vi "Fill FN - Post-Fill Wait (SubVI).vi"(0 "Signals IN":T2={"Dispense"=FALSE, "Fill"=FALSE, "Spray"=FALSE, "Drain"=TRUE, "Complete"=FALSE, "Fill Error"=FALSE, "Dispense Error"=FALSE, "Fill Timeout"=FALSE, "Dispense Timeout"=FALSE}, 1 "Values IN":T1 {"Drain Time (s)" format="%.2f"; "Drain Rate (g/sec)" format="%.2f"}, 2 "Measured Mass (g)":dbl(knob) scale=0.0..1000.0, 3 "Settings":T3={"ON Settings"={"Enable Dynamic Setpoint?"=TRUE, "Enable Dynamic Dispense Time?"=TRUE, "Enable Drain Rate Functions"=TRUE, "Dispense Sample Time (s)"=0.5, "Dispense Slope Ave"=0, "ON Timeout (sec)"=600.0, "1st Setpoint (% of Target)"=0.0, "2nd Setpoint (% of Target)"=0.0, "3rd Setpoint (% of Target)"=0.0, "Measure Dispense Delay (sec)"=0.0, "Settle Slope Sample Time (s)"=0.0}, "OFF Settings"={"Drain Sample Time (s)"=0.5, "Drain Rate Ave Size"=5, "Drain Rate Limits (± g/sec)"=10.0, "Level Slope Range (± g/sec)"=0.25, "OFF Timeout (sec)"=0.0, "Near SP Slope Level (± g/sec)"=0.01, "Near Setpoint Threshold (%)"=95.0}, "Overshoot Settings"={"Time Limit (s)"=60.0, "Container MAX (g)"=1500.0, "Max FILL Slope (+/- g/sec)"=10.0, "% Overshot to Enable (>)"=0.25}, "FILL Timeout (s)"=300.0, "Full Settle Time (s)"=20.0, "Pre-Hydrate \nSpray Time (s)"=10.0, "Pre-Hydrate \nWait Time (s)"=30.0}, 5 "Fill Case Change?":bool) -> (14 "Signals OUT":T2, 15 "Values OUT":T1, 19 "Case Complete":bool)   [LabVIEW 2012]
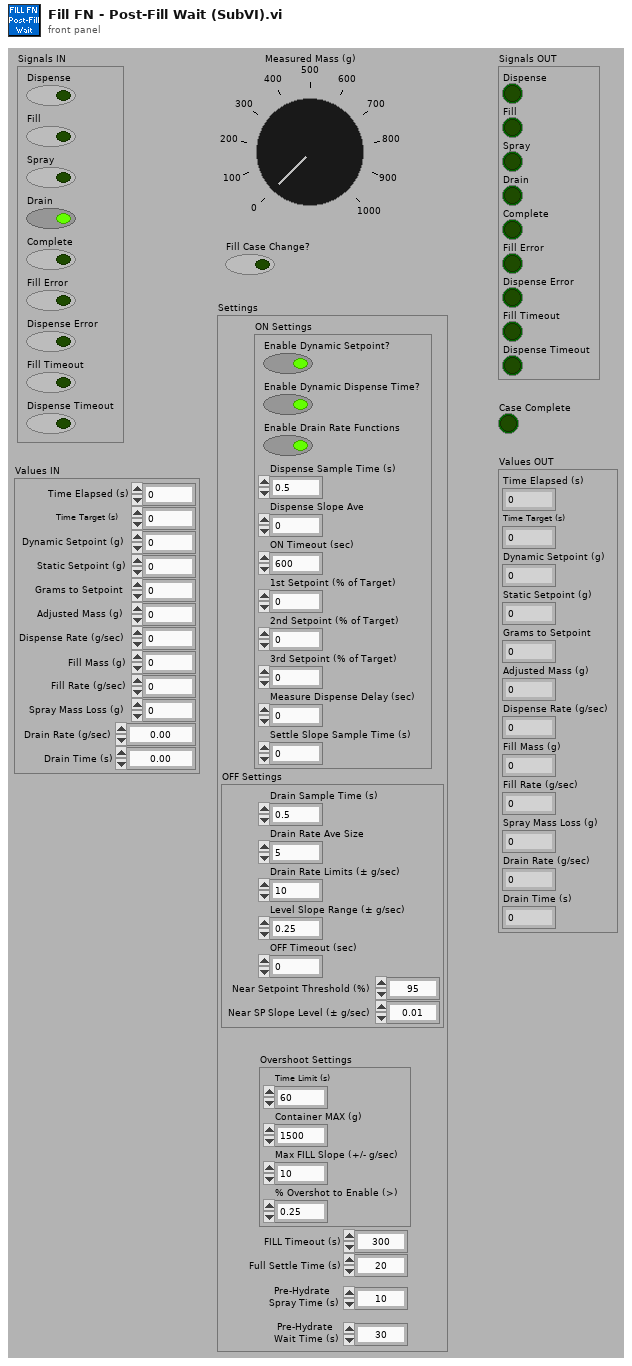
[diagram p1: front panel]
types:
  T1 = cluster{"Time Elapsed (s)":dbl, "Time Target (s)":dbl, "Dynamic Setpoint (g)":dbl, "Static Setpoint (g)":dbl, "Grams to Setpoint":dbl, "Adjusted Mass (g)":dbl, "Dispense Rate (g/sec)":dbl, "Fill Mass (g)":dbl, "Fill Rate (g/sec)":dbl, "Spray Mass Loss (g)":dbl, "Drain Rate (g/sec)":dbl, "Drain Time (s)":dbl}
  T2 = cluster{"Dispense":bool, "Fill":bool, "Spray":bool, "Drain":bool, "Complete":bool, "Fill Error":bool, "Dispense Error":bool, "Fill Timeout":bool, "Dispense Timeout":bool}
  T3 = cluster{"ON Settings":cluster{"Enable Dynamic Setpoint?":bool, "Enable Dynamic Dispense Time?":bool, "Enable Drain Rate Functions":bool, "Dispense Sample Time (s)":dbl, "Dispense Slope Ave":i32, "ON Timeout (sec)":dbl, "1st Setpoint (% of Target)":dbl, "2nd Setpoint (% of Target)":dbl, "3rd Setpoint (% of Target)":dbl, "Measure Dispense Delay (sec)":dbl, "Settle Slope Sample Time (s)":dbl}, "OFF Settings":cluster{"Drain Sample Time (s)":dbl, "Drain Rate Ave Size":i32, "Drain Rate Limits (± g/sec)":dbl, "Level Slope Range (± g/sec)":dbl, "OFF Timeout (sec)":dbl, "Near SP Slope Level (± g/sec)":dbl, "Near Setpoint Threshold (%)":dbl}, "Overshoot Settings":cluster{"Time Limit (s)":dbl, "Container MAX (g)":dbl, "Max FILL Slope (+/- g/sec)":dbl, "% Overshot to Enable (>)":dbl}, "FILL Timeout (s)":dbl, "Full Settle Time (s)":dbl, "Pre-Hydrate \nSpray Time (s)":dbl, "Pre-Hydrate \nWait Time (s)":dbl}
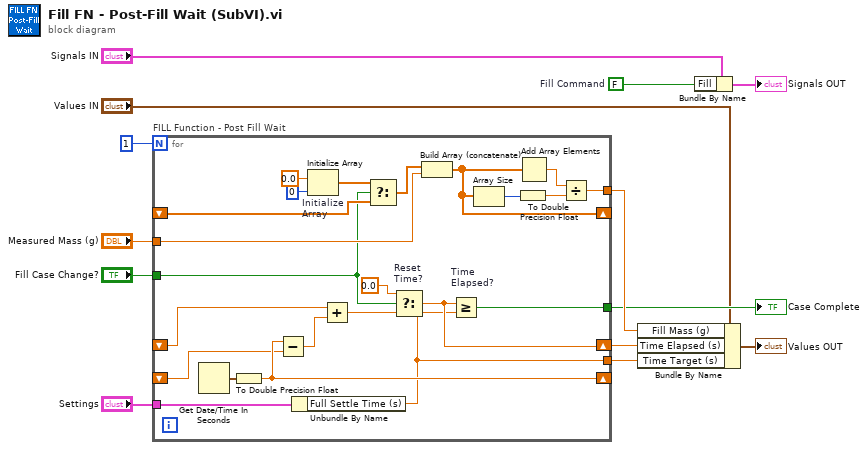
[diagram p0: block diagram]
diagram:
  w6 = FALSE  # Fill Command
  n1 = for "FILL Function - Post Fill Wait" {
    N: 1 -> [_]
    shift-right: [w35] -> _
    shift-left: _ -> [w34]
    shift-right: [w29] -> w9
    shift-left: _ -> [w32]
    tunnel: "Measured Mass (g)" -> [w19]
    tunnel: "Fill Case Change?" -> [w18]
    tunnel: [w17] -> w13
    shift-right: [w26] -> _
    shift-left: _ -> [w20]
    tunnel: [w14] -> w10
    tunnel: [w16] -> w11
    tunnel: "Settings" -> [w15]
    n2 = Get Date/Time In Seconds() -> (seconds since 1Jan1904=w36:timestamp)
    n3 = To Double Precision Float(number=w36) -> (double precision float=w35:dbl)
    n4 = Subtract(x=w35, y=w34) -> (x-y=w31:dbl)
    n5 = Unbundle By Name(w15) -> ("Full Settle Time (s)"=w14:dbl)
    n6 = Initialize Array "Initialize\nArray"(0.0 ("Measured Mass (g)"), 0 ("dimension size")) -> (w22:dbl[])
    n7 = Add(x=w32, y=w31) -> (x+y=w33:dbl)
    n8 = Select(t=w22, s=w18, f=w20) -> (s? t:f=w21:dbl[])
    n9 = Select "Reset\nTime?"(t=0.0, s=w18, f=w33) -> (s? t:f=w29:dbl)
    n10 = Build Array (concatenate)(w21, w19) -> (w26:dbl[])
    n11 = Greater Or Equal? "Time\nElapsed?"(x=w29, y=w14) -> (x >= y?=w16:bool)
    n12 = Array Size(array=w26) -> (size(s)=w24:i32)
    n13 = To Double Precision Float(number=w24) -> (double precision float=w23:dbl)
    n14 = Add Array Elements(numeric array=w26) -> (sum=w25:dbl)
    n15 = Divide(x=w25, y=w23) -> (x/y=w17:dbl)
  }
  "Case Complete" <- w11
  n16 = Bundle By Name(cluster="Values IN", "Fill Mass (g)"=w13, "Time Elapsed (s)"=w9, "Time Target (s)"=w10) -> (→"Values OUT":T1)
  n17 = Bundle By Name(cluster="Signals IN", "Fill"=w6) -> (→"Signals OUT":T2)
